vi "Text Description.vi"(11 "Message":refnum<class "MSG.lvclass">) -> (2 "Description":string, 3 "Message":refnum<class "MSG.lvclass">)   [LabVIEW 2011, in "Messenging.lvlib" / "MSG.lvclass"]
uses:
  MSG.lvclass
  Send/Send.lvclass
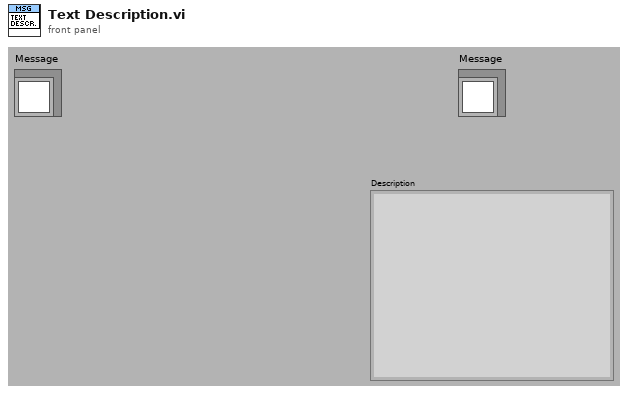
[diagram p1: front panel]
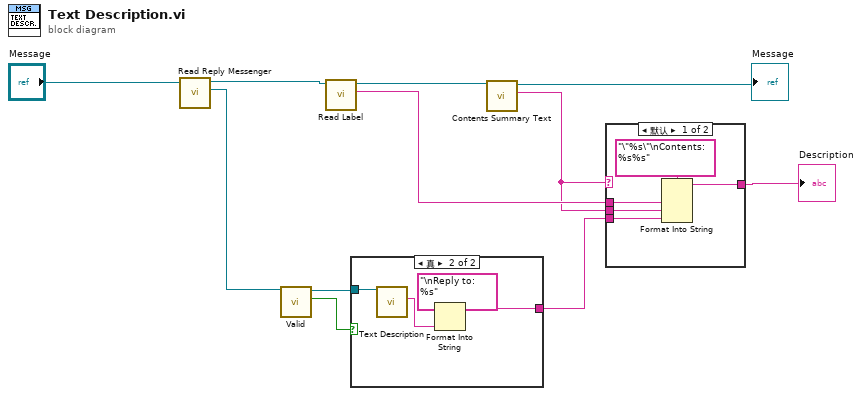
[diagram p0: block diagram]
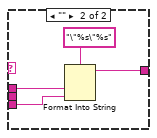
[diagram p2: hidden frame]
diagram:
  n1 = call-dynamic "Read Reply Messenger.vi"("Messege"="Message") -> ("Reply to..."=w10:refnum<class "Send.lvclass">, "Message"=w5:refnum<class "MSG.lvclass">)  [unwired: 1 in, 8 out]
  n2 = call-dynamic "Valid.vi"("Send in"=w10) -> ("Valid?"=w8:bool, "Send out"=w9:refnum<class "Send.lvclass">)  [unwired: 9 out]
  n3 = call-dynamic "Read Label.vi"("Message"=w5) -> ("Label"=w4:string, "Message"=w11:refnum<class "MSG.lvclass">)  [unwired: 1 in, 8 out]
  n4 = case shown="真" w8 {
    tunnel: [_ w14] -> w3
    tunnel: w9 -> [_ w13]
    frame False {
    }
    frame True {
      n5 = call-dynamic "Text Description.vi"("Send in"=w13) -> ("Description"=w12:string)  [unwired: 10 out]
      n6 = Format Into String(format string="\nReply to: %s", w12) -> (resulting string=w14:string)  [unwired: 2 in, 1 out]
    }
  }
  n7 = call-dynamic "Contents Summary Text.vi"("Message"=w11) -> ("Contents Summary Text"=w1:string, "Message"=→"Message":refnum<class "MSG.lvclass">)  [unwired: 9 out]
  n8 = case shown="默认" w1 {
    tunnel: w4 -> [w19 w23]
    tunnel: w1 -> [w18 _]
    tunnel: w3 -> [w17 w22]
    tunnel: [w16 w21] -> w2
    frame Default {
      n9 = Format Into String(format string="\"%s\"\nContents: %s%s", w19, w18, w17) -> (resulting string=w16:string)  [unwired: 2 in, 1 out]
    }
    frame "" {
      n10 = Format Into String(format string="\"%s\"%s", w23, w22) -> (resulting string=w21:string)  [unwired: 2 in, 1 out]
    }
  }
  "Description" <- w2
